vi "采配水UI.vi"() -> ()   [LabVIEW 2016, in "采配水.lvlib"]
uses:
  <vilib>/Utility/miscctls.llb/LVPointTypeDef.ctl
  <vilib>/Plasmionique/MB Master/MB_Master/MB_Master.lvclass
  <vilib>/Utility/config.llb/NI_LVConfig.lvlib
  <vilib>/ptbypt/NI_PtbyPt.lvlib
  AIRMAR WeatherCaster/AIRMAR WeatherCaster.lvlib
panel:
  in  "停止":bool
  out "运行状态":string
  in  "采配水单次启动":bool
  out "通讯状态":bool
  in  "采配水设置":bool caption="报警设置"
  in  "排液阀":bool
  in  "采水泵":bool
  out "液位状态":bool
  in  "ZLAN启用":bool
  # "监控信息"
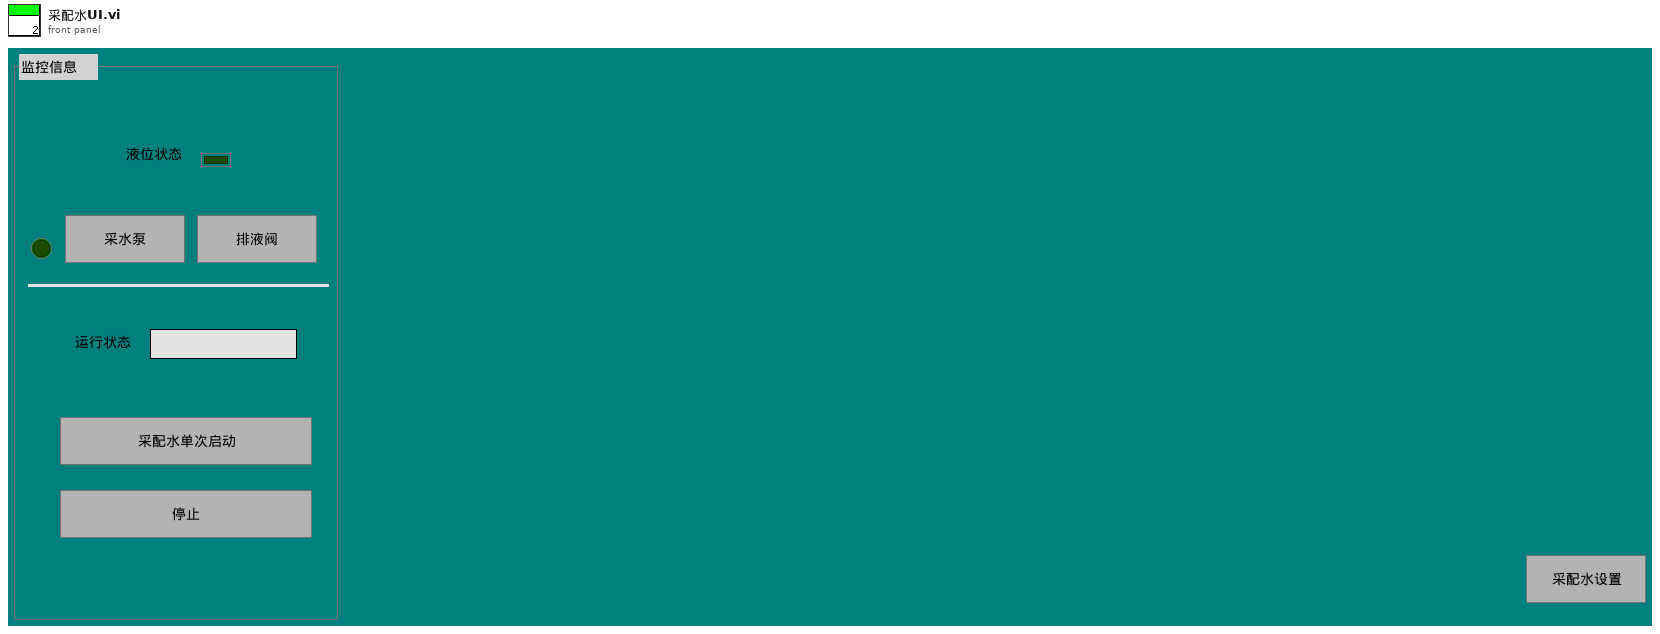
[diagram p1: front panel]
types:
  T1 = typedef "LVPointTypeDef.ctl" = cluster{"Horizontal":i16, "Vertical":i16}
  T2 = cluster{"蓄电池电压":dbl, "室温":dbl, "湿度":dbl, "水浸报警":bool, "烟雾报警":bool, "门禁1状态":bool, "门禁2状态":bool}
  T3 = cluster{"AD0":dbl, "AD1":dbl, "AD2":dbl, "AD3":dbl, "AD4":dbl, "AD5":dbl, "AD6":dbl, "AD7":dbl}
  T4 = cluster{"AD0":dbl, "AD1":dbl, "AD1":dbl, "AD3":dbl, "AD4":dbl, "AD5":dbl, "AD6":dbl, "AD7":dbl}
  T5 = cluster{"环境变量":cluster{"蓄电池电压":dbl, "室温":dbl, "湿度":dbl, "水浸报警":bool, "烟雾报警":bool, "门禁1状态":bool, "门禁2状态":bool}, "ZLAN 6842 MB session":refnum<class "MB_Master.lvclass">, "DI":bool[], "DO":bool[]}
  T6 = typedef "NI_LVConfig.lvlib/Config Data RefNum.ctl" = refnum<k1>
  T7 = cluster{"Registers[0]":u16, "Registers[1]":u16, "Registers[2]":u16, "Registers[3]":u16, "Registers[4]":u16, "Registers[5]":u16, "Registers[6]":u16, "Registers[7]":u16}
  T8 = enum32{"Bad", "Idle", "Run top level", "Running"}
  T9 = cluster{"排空时间":dbl, "润洗时间":dbl, "进样超时时间":dbl, "沉淀时间":dbl, "配水时间":dbl}
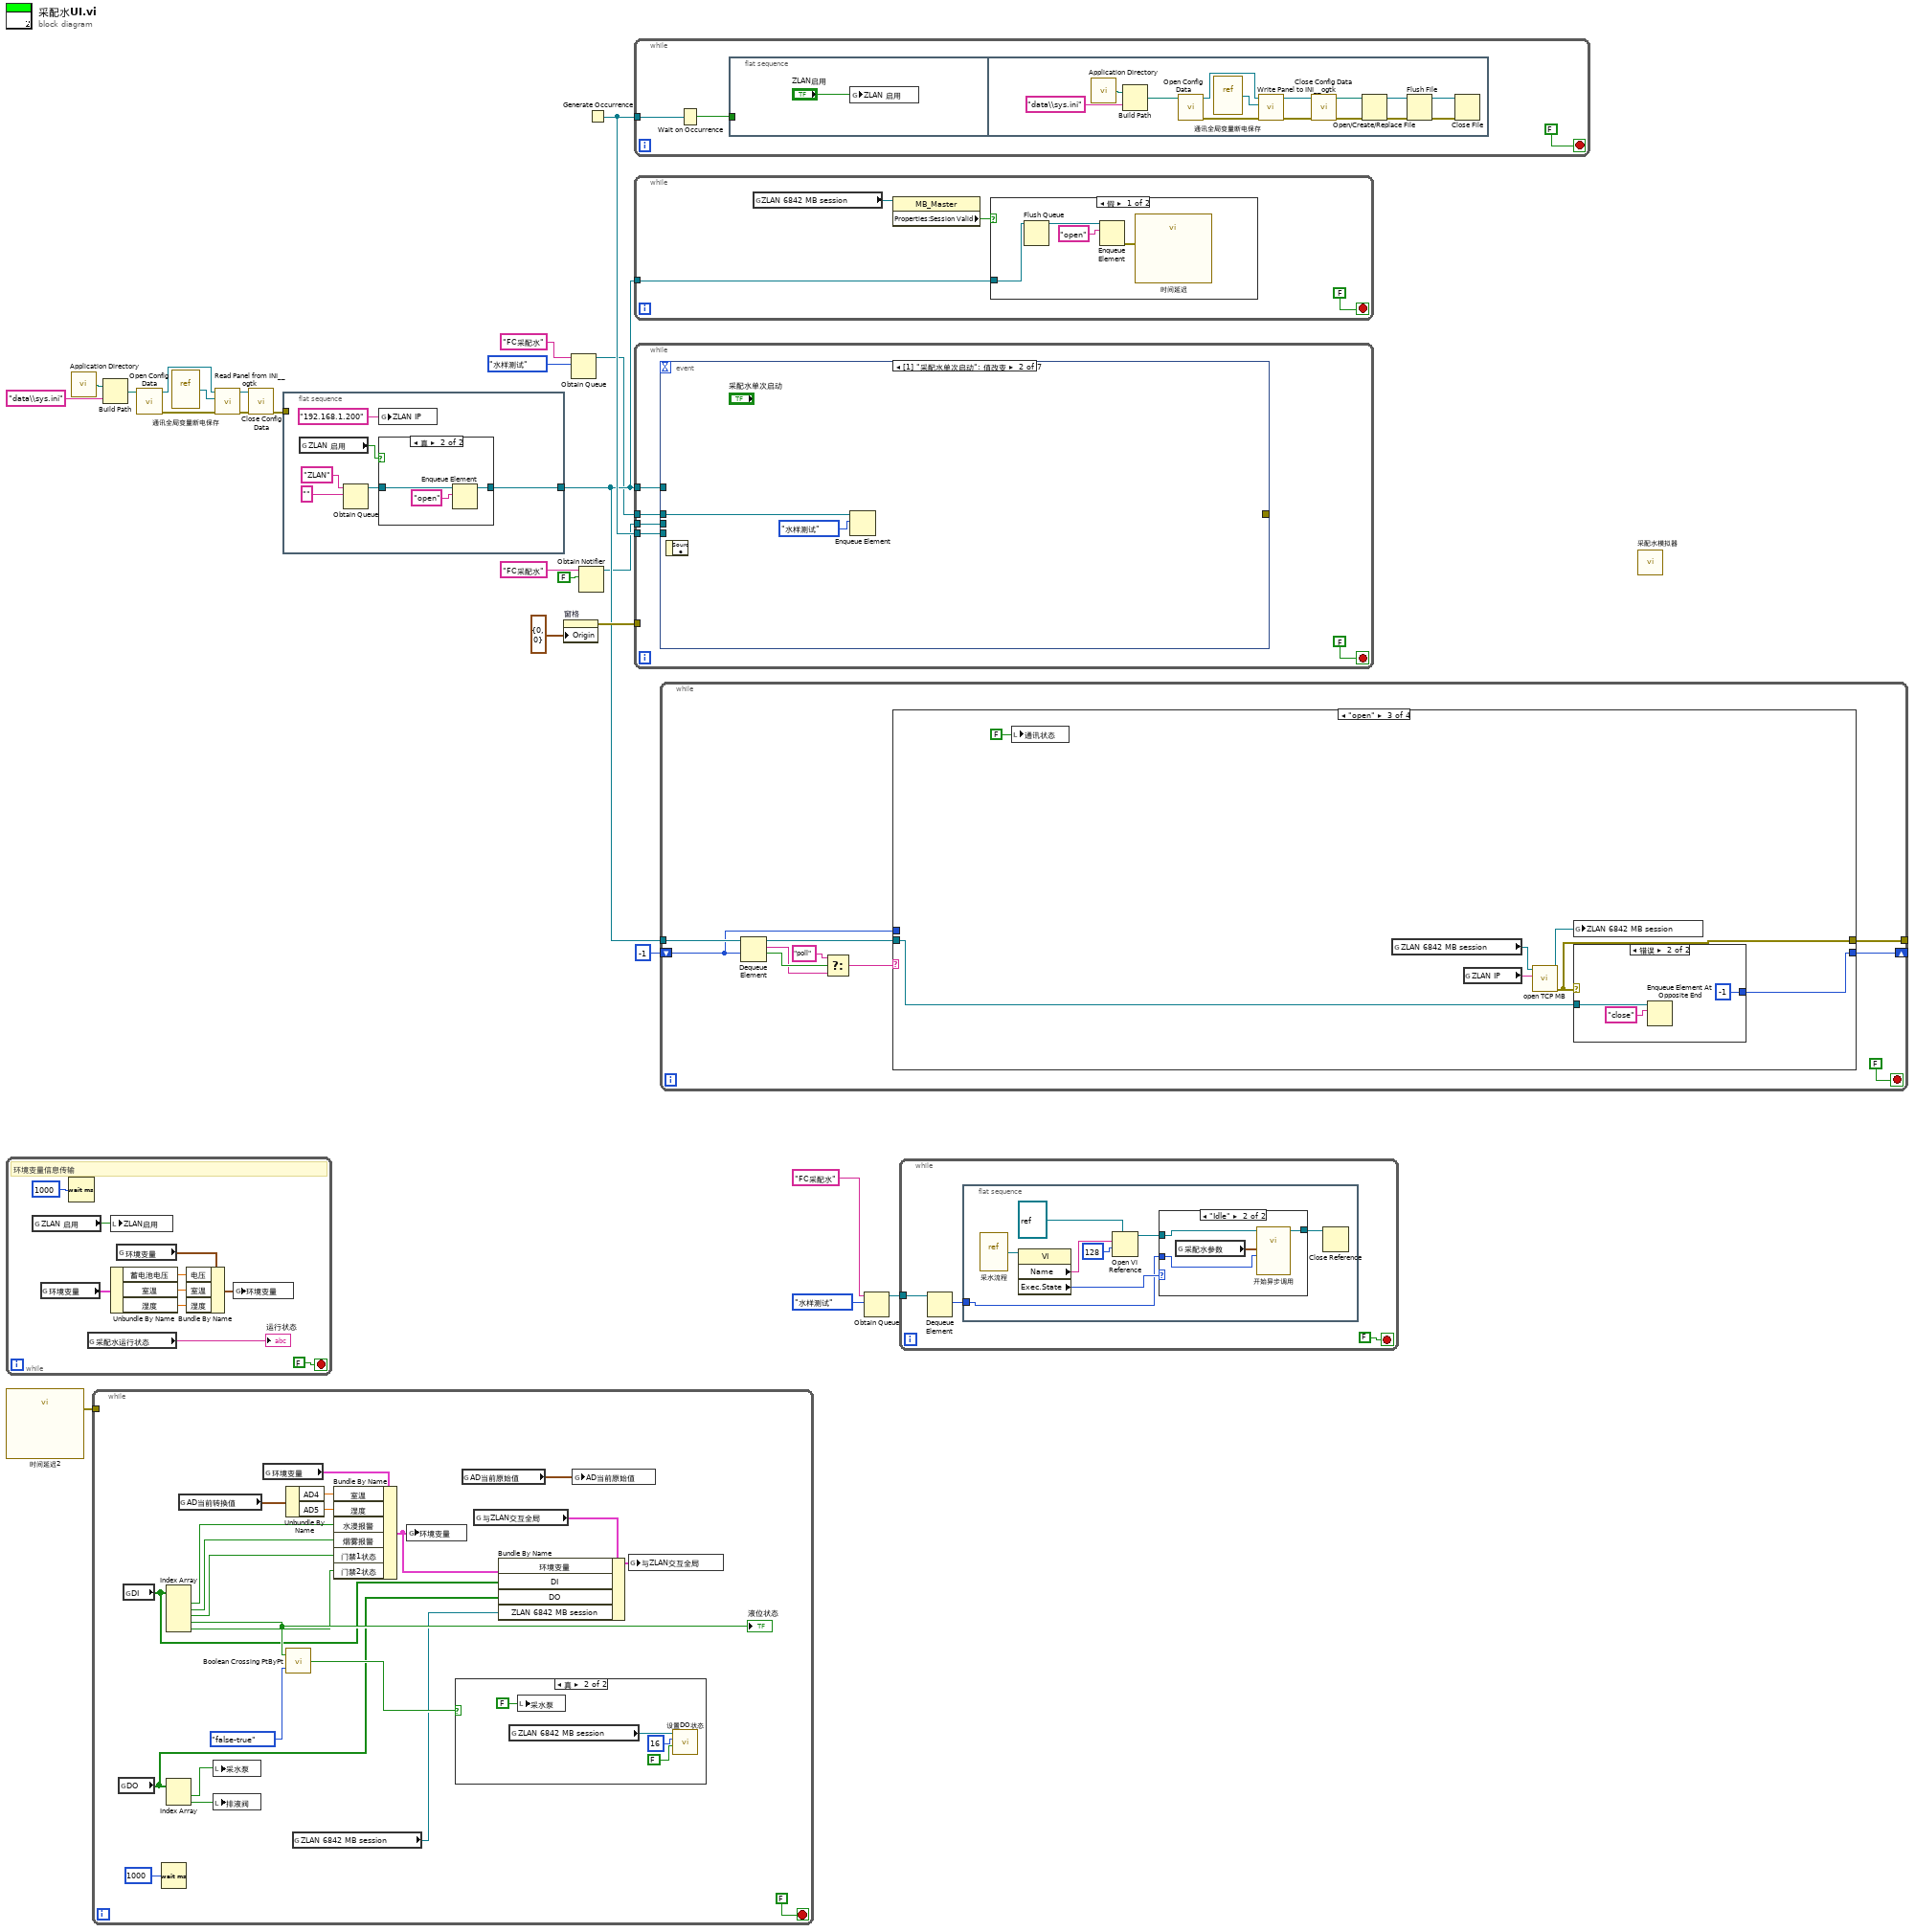
[diagram p0: block diagram]
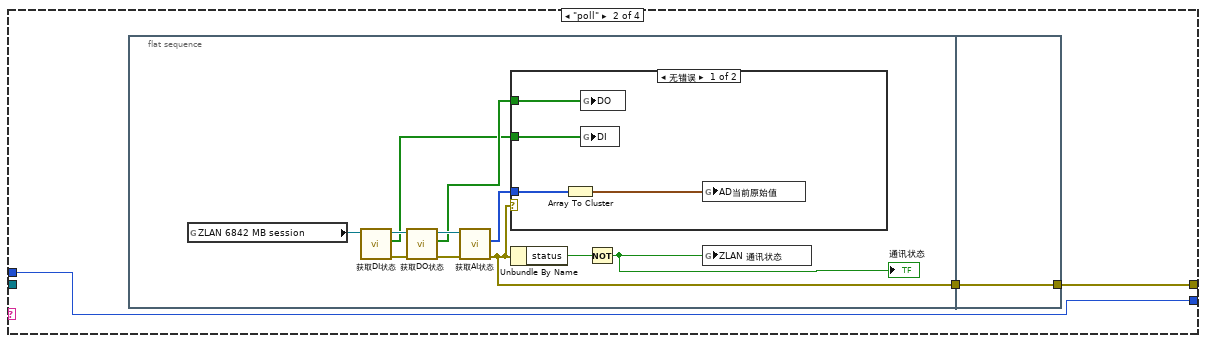
[diagram p7: hidden frame]
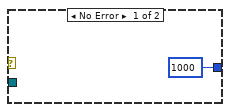
[diagram p9: hidden frame]
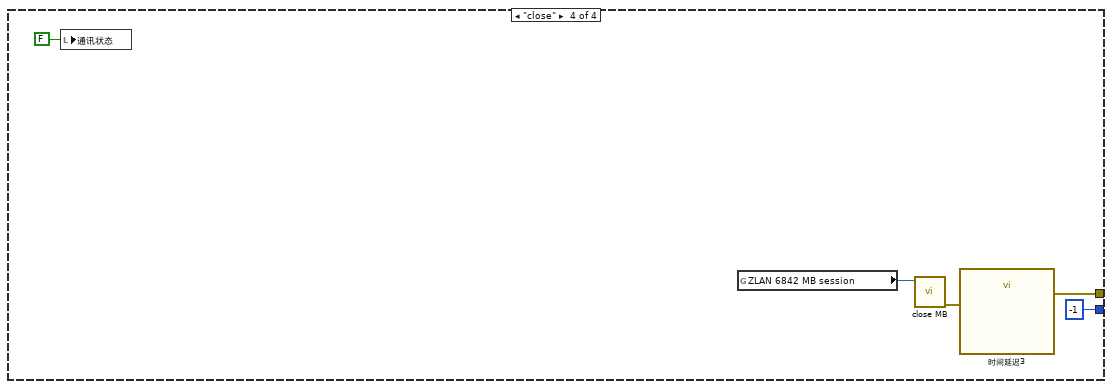
[diagram p10: hidden frame]
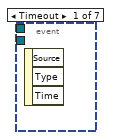
[diagram p11: hidden frame]
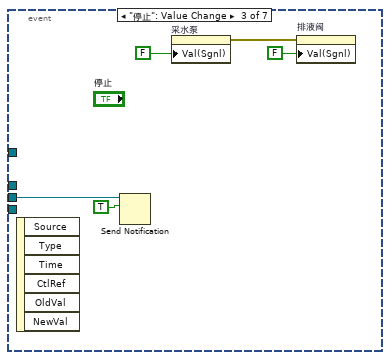
[diagram p12: hidden frame]
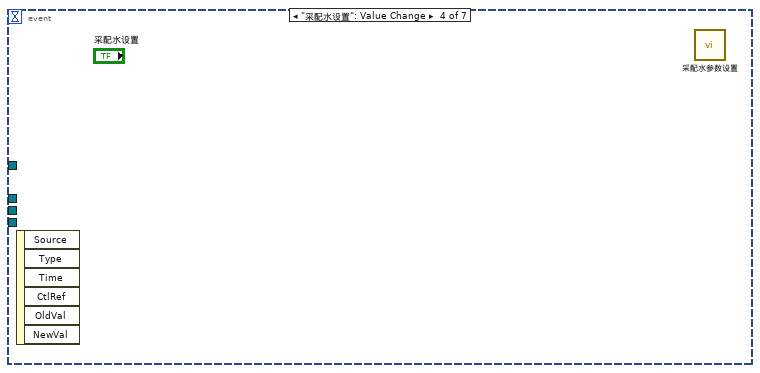
[diagram p13: hidden frame]
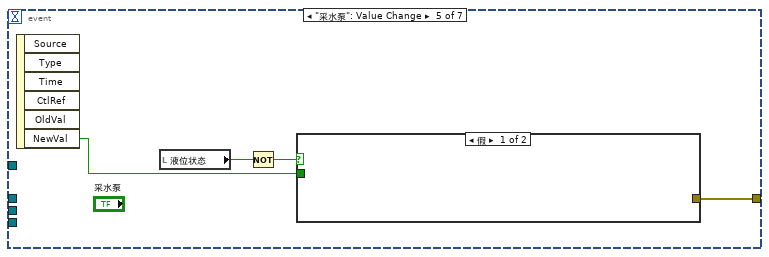
[diagram p14: hidden frame]
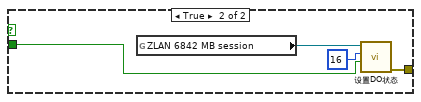
[diagram p15: hidden frame]
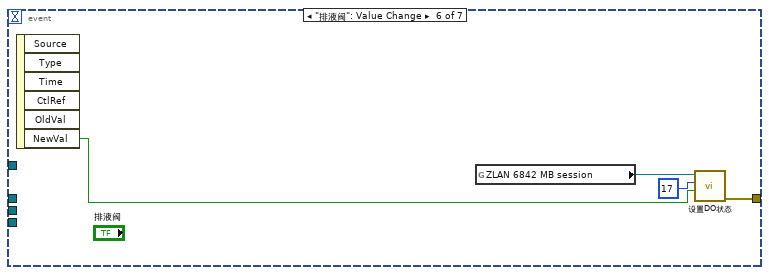
[diagram p16: hidden frame]
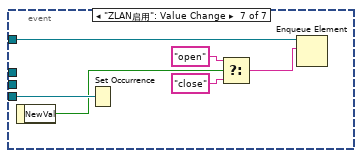
[diagram p17: hidden frame]
diagram:
  n1 = while {
    stop <- FALSE stop-if-true
    # "环境变量信息传输"
    n2 = global read "通讯全局变量断电保存.vi" "ZLAN 启用"() -> (w26:bool)
    n3 = global read "通讯全局变量.vi" "环境变量"() -> (w31:T2)
    n4 = Wait (ms)(milliseconds to wait=u32 1000 ("等待时间（毫秒）")) -> ()  [unwired: 1 out]
    n5 = global read "通讯全局变量.vi" "采配水运行状态"() -> (→"运行状态":string)
    n6 = local write "ZLAN启用"(w26) -> ()
    n7 = Unbundle By Name(w31) -> ("蓄电池电压"=w30:dbl, "室温"=w29:dbl, "湿度"=w28:dbl)
    n8 = global read "气象全局变量.vi" "环境变量"() -> (w32:cluster{"电压":dbl, "室温":dbl, "湿度":dbl})
    n9 = Bundle By Name(cluster=w32, "电压"=w30, "室温"=w29, "湿度"=w28) -> (w33:cluster{"电压":dbl, "室温":dbl, "湿度":dbl})
    n10 = global write "气象全局变量.vi" "环境变量"(w33) -> ()
  }
  n11 = call "时间延迟2"() -> ("error out"=w14:errorcluster)  [unwired: 11 in]
  n12 = call <vilib>:"Application Directory.vi"() -> ("Application Directory"=w16:path)
  n13 = while {
    tunnel: w14 -> [_]
    stop <- FALSE stop-if-true
    n14 = global read "通讯全局变量.vi" "DO"() -> (w38:bool[])
    n15 = global read "通讯全局变量.vi" "DI"() -> (w39:bool[])
    n16 = Wait (ms)(milliseconds to wait=u32 1000 ("等待时间（毫秒）")) -> ()  [unwired: 1 out]
    n17 = Index Array(array=w39) -> (element #1=w48:bool, element #2=w47:bool, element #3=w46:bool, element #4=w52:bool, element #5=w45:bool)  [unwired: 5 in]
    "液位状态" <- w52
    n18 = Index Array(array=w38) -> (element #1=w54:bool, element #2=w53:bool)  [unwired: 2 in]
    n19 = global read "断电保存全局变量.vi" "AD当前转换值"() -> (w35:T3)
    n20 = local write "采水泵"(w54) -> ()
    n21 = local write "排液阀"(w53) -> ()
    n22 = global read "通讯全局变量.vi" "环境变量"() -> (w49:T2)
    n23 = Unbundle By Name(w35) -> ("AD4"=w44:dbl, "AD5"=w43:dbl)
    n24 = call <vilib>:"Boolean Crossing PtByPt.vi"("direction"=enum16{"either", "false-true", "true-false"}."false-true", "input"=w52) -> ("crossing"=w51:bool)  [unwired: 1 in]
    n25 = global read "通讯全局变量.vi" "ZLAN 6842 MB session"() -> (w37:refnum<class "MB_Master.lvclass">)
    n26 = Bundle By Name(cluster=w49, "室温"=w44, "湿度"=w43, "水浸报警"=w48, "烟雾报警"=w47, "门禁1状态"=w46, "门禁2状态"=w45) -> (w40:T2)
    n27 = global write "通讯全局变量.vi" "环境变量"(w40) -> ()
    n28 = case shown="真" w51 {
      frame False {
      }
      frame True {
        n29 = global read "通讯全局变量.vi" "ZLAN 6842 MB session"() -> (w60:refnum<class "MB_Master.lvclass">)
        n30 = local write "采水泵"(FALSE ("采水泵")) -> ()
        n31 = call "设置DO状态.vi"("value"=FALSE, "address"=u16 16, "MB session in"=w60) -> ()  [unwired: 7 in, 2 out]
      }
    }
    n32 = global read "通讯全局变量.vi" "AD当前原始值"() -> (w36:T4)
    n33 = global read "外部交互全局变量.vi" "与ZLAN交互全局"() -> (w42:T5)
    n34 = Bundle By Name(cluster=w42, "环境变量"=w40, "DI"=w39, "DO"=w38, "ZLAN 6842 MB session"=w37) -> (w41:T5)
    n35 = global write "断电保存全局变量.vi" "AD当前原始值"(w36) -> ()
    n36 = global write "外部交互全局变量.vi" "与ZLAN交互全局"(w41) -> ()
  }
  n37 = Build Path(base path=w16, name or relative path="data\\sys.ini" ("名称或相对路径")) -> (appended path=w18:path)
  n38 = call <vilib>:"Open Config Data.vi"("configuration file path"=w18) -> ("error out"=w22:errorcluster, "refnum"=w19:T6)  [unwired: 8 in, 1 out]
  n39 = vi-ref "通讯全局变量断电保存.vi"() -> (w20:refnum<vi>)
  n40 = call <userlib>:"Read Panel from INI__ogtk.vi"("error in (no error)"=w22, "VI ref"=w20, "refnum"=w19) -> ("error out"=w15:errorcluster, "refnum out"=w21:T6)  [unwired: 7 in]
  n41 = call <vilib>:"Close Config Data.vi"("error in (no error)"=w15, "refnum"=w21) -> ("error out"=w11:errorcluster)  [unwired: 8 in, 1 out]
  n42 = flat-sequence {
    tunnel: [w63] -> w10
    tunnel: w11 -> [_]
    frame #0 {
      n43 = global read "通讯全局变量断电保存.vi" "ZLAN 启用"() -> (w62:bool)
      n44 = Obtain Queue(name (unnamed)="ZLAN" ("名称（未命名）"), element data type="") -> (queue out=w64:refnum<queue>)  [unwired: 3 in, 2 out]
      n45 = global write "通讯全局变量断电保存.vi" "ZLAN IP"("192.168.1.200" ("ZLAN IP")) -> ()
      n46 = case shown="真" w62 {
        tunnel: w64 -> [w67 w70]
        tunnel: [w67 w68] -> w63
        frame False {
        }
        frame True {
          n47 = Enqueue Element(queue=w70, element="open" ("元素")) -> (queue out=w68:refnum<queue>)  [unwired: 2 in, 2 out]
        }
      }
    }
  }
  n48 = property on="窗格" class="Pane"("Origin"=T1 {"Horizontal"=0, "Vertical"=0} ("原点")) -> (error out=w23:errorcluster)  [unwired: 2 in, 1 out]
  n49 = Obtain Queue(name (unnamed)="FC采配水" ("名称（未命名）"), element data type=enum16{"水样测试", "加标回收"}."水样测试" ("启动类型")) -> (queue out=w4:refnum<queue>)  [unwired: 3 in, 2 out]
  n50 = Obtain Notifier(name (unnamed)="FC采配水" ("名称（未命名）"), notification data type=FALSE) -> (notifier out=w7:refnum<notifier>)  [unwired: 2 in, 2 out]
  n51 = Generate Occurrence() -> (w12:refnum<k4>)
  n52 = while {
    tunnel: w12 -> [w72]
    stop <- FALSE stop-if-true
    n53 = Wait on Occurrence(2:w72) -> (0:w71:bool)  [unwired: 2 in]
    n54 = flat-sequence {
      tunnel: w71 -> [_]
      frame #0 {
        n55 = global write "通讯全局变量断电保存.vi" "ZLAN 启用"("ZLAN启用") -> ()
      }
      frame #1 {
        n56 = call <vilib>:"Application Directory.vi"() -> ("Application Directory"=w88:path)
        n57 = Build Path(base path=w88, name or relative path="data\\sys.ini" ("名称或相对路径")) -> (appended path=w86:path)
        n58 = call <vilib>:"Open Config Data.vi"("configuration file path"=w86) -> ("error out"=w82:errorcluster, "refnum"=w85:T6)  [unwired: 8 in, 1 out]
        n59 = vi-ref "通讯全局变量断电保存.vi"() -> (w84:refnum<vi>)
        n60 = call <userlib>:"Write Panel to INI__ogtk.vi"("error in (no error)"=w82, "VI ref"=w84, "refnum"=w85) -> ("error out"=w81:errorcluster, "refnum out"=w83:T6)  [unwired: 7 in]
        n61 = call <vilib>:"Close Config Data.vi"("error in (no error)"=w81, "refnum"=w83) -> ("error out"=w76:errorcluster, "file path"=w75:path)  [unwired: 8 in]
        n62 = Open/Create/Replace File(file path (use dialog)=w75, error in=w76) -> (refnum out=w79:refnum<file>, error out=w80:errorcluster)  [unwired: 4 in, 1 out]
        n63 = Flush File(refnum=w79, error in=w80) -> (refnum out=w78:refnum<file>, error out=w77:errorcluster)
        n64 = Close File(refnum=w78, error in=w77) -> ()  [unwired: 2 out]
      }
    }
  }
  n65 = while {
    tunnel: w10 -> [w90]
    stop <- FALSE stop-if-true
    n66 = global read "通讯全局变量.vi" "ZLAN 6842 MB session"() -> (w92:refnum<class "MB_Master.lvclass">)
    n67 = property class="MB_Master"(reference=w92) -> ("Properties:Session Valid"=w91:bool)  [unwired: 1 in, 2 out]
    n68 = case shown="假" w91 {
      tunnel: w90 -> [w96 _]
      frame False {
        n69 = Flush Queue(queue=w96) -> (queue out=w95:refnum<queue>)  [unwired: 1 in, 2 out]
        n70 = Enqueue Element(queue=w95, element="open") -> (error out=w93:errorcluster)  [unwired: 2 in, 2 out]
        n71 = call "时间延迟"("error in (no error)"=w93) -> ()  [unwired: 10 in, 1 out]
      }
      frame True {
      }
    }
  }
  n72 = while {
    tunnel: w23 -> [_]
    tunnel: w10 -> [w100]
    tunnel: w12 -> [w99]
    tunnel: w7 -> [w98]
    tunnel: w4 -> [w97]
    stop <- FALSE stop-if-true
    n73 = event shown="[1] \"采配水单次启动\": 值改变" {
      selector: _ -> [_ _ _ _ _ _ _]
      dyn-events: _ -> [_ _ _ _ _ _ _]
      timeout: _ -> [_ _ _ _ _ _ _]
      tunnel: w100 -> [_ _ _ _ _ _ w124]
      tunnel: w99 -> [_ _ _ _ _ _ w126]
      tunnel: [_ _ _ _ w111 w117 _] -> _
      tunnel: w98 -> [_ _ w108 _ _ _ _]
      tunnel: w97 -> [_ w103 _ _ _ _ _]
      event Timeout {
        n74 = event-data() -> ()  [unwired: 1 in, 3 out]
      }
      event "采配水单次启动": Value Change {
        n75 = event-data() -> ()  [unwired: 1 in, 1 out]
        n76 = Enqueue Element(queue=w103, element=enum16{"水样测试", "加标回收"}."水样测试" ("元素")) -> ()  [unwired: 2 in, 3 out]
      }
      event "停止": Value Change {
        n77 = event-data() -> ()  [unwired: 1 in, 6 out]
        n78 = Send Notification(notification=TRUE ("通知"), notifier=w108) -> ()  [unwired: 1 in, 2 out]
        n79 = property on="采水泵" class="Bool (严格)"("Val(Sgnl)"=FALSE ("值(信号)")) -> (error out=w105:errorcluster)  [unwired: 2 in, 1 out]
        n80 = property on="排液阀" class="Bool (严格)"(error in=w105, "Val(Sgnl)"=FALSE ("值(信号)")) -> ()  [unwired: 1 in, 2 out]
      }
      event "采配水设置": Value Change {
        n81 = event-data() -> ()  [unwired: 1 in, 6 out]
        n82 = call "采配水参数设置.vi"() -> ()  [unwired: 12 in]
      }
      event "采水泵": Value Change {
        n83 = event-data() -> ("NewVal"=w112:bool)  [unwired: 1 in, 5 out]
        n84 = local read "液位状态"() -> (w109:bool)
        n85 = Not(x=w109) -> (.not. x?=w110:bool)
        n86 = case shown="假" w110 {
          tunnel: w112 -> [_ w114]
          tunnel: [_ w113] -> w111
          frame False {
          }
          frame True {
            n87 = global read "通讯全局变量.vi" "ZLAN 6842 MB session"() -> (w116:refnum<class "MB_Master.lvclass">)
            n88 = call "设置DO状态.vi"("value"=w114, "address"=u16 16, "MB session in"=w116) -> ("error out"=w113:errorcluster)  [unwired: 7 in, 1 out]
          }
        }
      }
      event "排液阀": Value Change {
        n89 = event-data() -> ("NewVal"=w118:bool)  [unwired: 1 in, 5 out]
        n90 = global read "通讯全局变量.vi" "ZLAN 6842 MB session"() -> (w120:refnum<class "MB_Master.lvclass">)
        n91 = call "设置DO状态.vi"("value"=w118, "address"=u16 17, "MB session in"=w120) -> ("error out"=w117:errorcluster)  [unwired: 7 in, 1 out]
      }
      event "ZLAN启用": Value Change {
        n92 = event-data() -> ("NewVal"=w125:bool)  [unwired: 1 in]
        n93 = Set Occurrence(w126) -> ()
        n94 = Select(t="open", s=w125, f="close") -> (s? t:f=w122:string)
        n95 = Enqueue Element(queue=w124, element=w122) -> ()  [unwired: 2 in, 3 out]
      }
    }
  }
  n96 = while {
    tunnel: w10 -> [w136]
    tunnel: [w128] -> _
    shift-right: [w129] -> _
    shift-left: -1 ("超时毫秒(-1)") -> [w130]
    stop <- FALSE stop-if-true
    n97 = Dequeue Element(queue=w136, timeout in ms (-1)=w130) -> (queue out=w127:refnum<queue>, element=w133:string, timed out?=w135:bool)  [unwired: 1 in, 1 out]
    n98 = Select(t="poll" ("元素"), s=w135, f=w133) -> (s? t:f=w132:string)
    n99 = case shown="\"open\"" w132 {
      tunnel: [_ w140 w159 w168] -> w128
      tunnel: w130 -> [w137 w138 _ _]
      tunnel: [w137 w138 w157 -1 ("超时毫秒(-1)")] -> w129
      tunnel: w127 -> [_ _ w158 _]
      frame Default {
      }
      frame "poll" {
        n100 = flat-sequence {
          tunnel: [w149] -> w139
          tunnel: [w156] -> w140
          tunnel: w139 -> [w156]
          frame #0 {
            n101 = global read "通讯全局变量.vi" "ZLAN 6842 MB session"() -> (w148:refnum<class "MB_Master.lvclass">)
            n102 = call "获取DI状态.vi"("MB session in"=w148) -> ("error out"=w146:errorcluster, "Coils"=w142:bool[], "MB session out"=w147:refnum<class "MB_Master.lvclass">)  [unwired: 8 in]
            n103 = call "获取DO状态.vi"("error in (no error)"=w146, "MB session in"=w147) -> ("error out"=w145:errorcluster, "Coils"=w143:bool[], "MB session out"=w144:refnum<class "MB_Master.lvclass">)  [unwired: 7 in]
            n104 = call "获取AI状态.vi"("error in (no error)"=w145, "MB session in"=w144) -> ("error out"=w149:errorcluster, "Registers"=w151:u16[])  [unwired: 7 in, 1 out]
            n105 = case shown="无错误" w149 {
              tunnel: w151 -> [w154 _]
              tunnel: w143 -> [w153 _]
              tunnel: w142 -> [w152 _]
              frame No Error {
                n106 = Array To Cluster(array=w154) -> (cluster=w155:T7)
                n107 = global write "通讯全局变量.vi" "DO"(w153) -> ()
                n108 = global write "通讯全局变量.vi" "DI"(w152) -> ()
                n109 = global write "通讯全局变量.vi" "AD当前原始值"(w155) -> ()
              }
              frame Error {
              }
            }
            n110 = Unbundle By Name(w149) -> ("status"=w150:bool)
            n111 = Not(x=w150) -> (.not. x?=w141:bool)
            "通讯状态" <- w141
            n112 = global write "通讯全局变量.vi" "ZLAN 通讯状态"(w141) -> ()
          }
          frame #1 {
          }
        }
      }
      frame "open" {
        n113 = local write "通讯状态"(FALSE ("通讯状态")) -> ()
        n114 = global read "通讯全局变量.vi" "ZLAN 6842 MB session"() -> (w162:refnum<class "MB_Master.lvclass">)
        n115 = global read "通讯全局变量断电保存.vi" "ZLAN IP"() -> (w160:string)
        n116 = call "open TCP MB.vi"("IP Address"=w160, "MB session in"=w162) -> ("error out"=w159:errorcluster, "MB session out"=w161:refnum<class "MB_Master.lvclass">)  [unwired: 8 in]
        n117 = global write "通讯全局变量.vi" "ZLAN 6842 MB session"(w161) -> ()
        n118 = case shown="错误" w159 {
          tunnel: w158 -> [_ w167]
          tunnel: [1000 ("超时毫秒(-1)") -1 ("超时毫秒(-1)")] -> w157
          frame No Error {
          }
          frame Error {
            n119 = Enqueue Element At Opposite End(queue=w167, element="close" ("元素")) -> ()  [unwired: 2 in, 3 out]
          }
        }
      }
      frame "close" {
        n120 = local write "通讯状态"(FALSE ("通讯状态")) -> ()
        n121 = global read "通讯全局变量.vi" "ZLAN 6842 MB session"() -> (w170:refnum<class "MB_Master.lvclass">)
        n122 = call "close MB.vi"("MB session in"=w170) -> ("error out"=w169:errorcluster)  [unwired: 10 in]
        n123 = call "时间延迟3"("error in (no error)"=w169) -> ("error out"=w168:errorcluster)  [unwired: 10 in]
      }
    }
  }
  n124 = Obtain Queue(name (unnamed)="FC采配水" ("名称（未命名）"), element data type=enum16{"水样测试", "加标回收"}."水样测试" ("启动类型")) -> (queue out=w1:refnum<queue>)  [unwired: 3 in, 2 out]
  n125 = while {
    tunnel: w1 -> [w174]
    stop <- FALSE stop-if-true
    n126 = Dequeue Element(queue=w174) -> (element=w173:enum16{"水样测试", "加标回收"})  [unwired: 2 in, 3 out]
    n127 = flat-sequence {
      tunnel: w173 -> [w176]
      frame #0 {
        n128 = vi-ref "采水流程.vi"() -> (w183:refnum<vi>)
        n129 = property class="VI"(reference=w183) -> ("Name"=w179:string, "Exec.State"=w181:T8)  [unwired: 1 in, 2 out]
        n130 = Open VI Reference(type specifier VI Refnum (for type only)=refnum<vi> refnum, vi path=w179, options=128 ("选项")) -> (vi reference=w178:refnum<vi>)  [unwired: 3 in, 1 out]
        n131 = case shown="\"Idle\"" w181 {
          tunnel: [w184 w188] -> w182
          tunnel: w178 -> [w184 w187]
          tunnel: w176 -> [_ w186]
          frame "Bad", Default {
          }
          frame "Idle" {
            n132 = global read "通讯全局变量断电保存.vi" "采配水参数"() -> (w185:T9)
            n133 = call-by-ref "开始异步调用"(reference=w187, "启动类型"=w186, "采配水参数"=w185) -> (reference out=w188:refnum<vi>)  [unwired: 11 in, 1 out]
          }
        }
        n134 = Close Reference(reference=w182) -> ()  [unwired: 1 in, 1 out]
      }
    }
  }
  n135 = call "采配水模拟器.vi"() -> ()  [unwired: 12 in]
